vi "Robotics Environment Simulator.vi"() -> ()   [LabVIEW 2011]
doc: "This VI starts and stops the environment simulator and serves as the master VI for your simulation code. Open and run this VI to display the environment simulator, or open the block diagram to view or modify simulation code."
uses:
  <vilib>/robotics/Simulator/NI_Robotics_Simulator.lvlib
panel:
  in  "manifest filename":string="Robotics Environment Simulator.xml"
  in  "stop":bool
  # "* Press the Run button to display the Robotics Environment Simulator.\n* Select Window>>Show Block Diagram or press <Ctrl-E> to view the block diagram, where you can add or modify simulation code. Add controls and indicators to the front panel of this VI to pass data into and out of the simulation code.\n* The manifest file must exist in same directory as the .lvproj file."
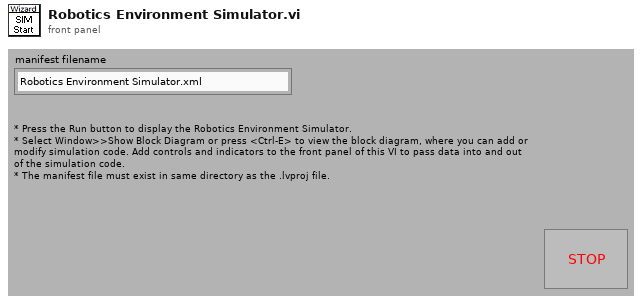
[diagram p1: front panel]
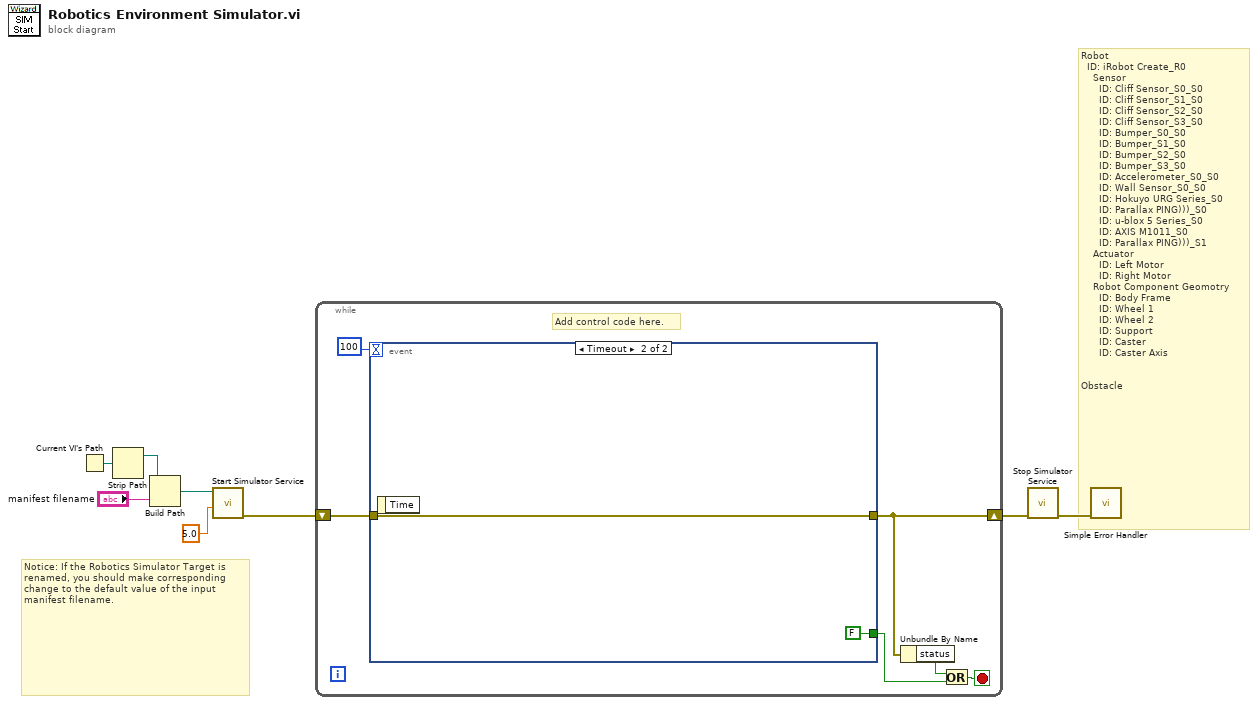
[diagram p0: block diagram]
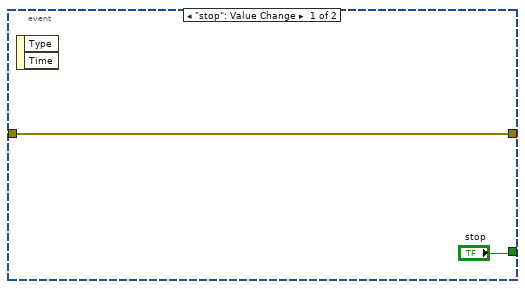
[diagram p2: hidden frame]
diagram:
  # "Robot\n\t\tID: iRobot Create_R0\n\t\t\t\tSensor\n\t\t\t\t\t\tID: Cliff Sensor_S0_S0\n\t\t\t\t\t\tID: Cliff Sensor_S1_S0\n\t\t\t\t\t\tID: Cliff Sensor_S2_S0\n\t\t\t\t\t\tID: Cliff Sensor_S3_S0\n\t\t\t\t\t\tID: Bumper_S0_S0\n\t\t\t\t\t\tID: Bumper_S1_S0\n\t\t\t\t\t\tID: Bumper_S2_S0\n\t\t\t\t\t\tID: Bumper_S3_S0\n\t\t\t\t\t\tID: Accelerometer_S0_S0\n\t\t\t\t\t\tID: Wall Sensor_S0_S0\n\t\t\t\t\t\tID: Hokuyo URG Series_S0\n\t\t\t\t\t\tID: Parallax PING)))_S0\n\t\t\t\t\t\tID: u-blox 5 Series_S0\n\t\t\t\t\t\tID: AXIS M1011_S0\n\t\t\t\t\t\tID: Parallax PING)))_S1\n\t\t\t\tActuator\n\t\t\t\t\t\tID: Left Motor\n\t\t\t\t\t\tID: Right Motor\n\t\t\t\tRobot Component Geomotry\n\t\t\t\t\t\tID: Body Frame\n\t\t\t\t\t\tID: Wheel 1\n\t\t\t\t\t\tID: Wheel 2\n\t\t\t\t\t\tID: Support\n\t\t\t\t\t\tID: Caster\n\t\t\t\t\t\tID: Caster Axis\n\n\nObstacle"
  # "Notice: If the Robotics Simulator Target is renamed, you should make corresponding change to the default value of the input manifest filename."
  n1 = Current VI's Path() -> (path=w6:path)
  n2 = Strip Path(path=w6) -> (stripped path=w5:path)  [unwired: 1 out]
  n3 = Build Path(base path=w5, name or relative path="manifest filename") -> (appended path=w4:path)
  n4 = call <vilib>:"Start Simulator Service.vi"("step size (ms)"=5.0 ("stepsize(ms)"), "manifest file"=w4) -> ("error out"=w1:errorcluster)  [unwired: 9 in]
  n5 = while {
    shift-right: [w10] -> w7
    shift-left: w1 -> [w13]
    stop <- w11 stop-if-true
    # "Add control code here."
    n6 = event shown="[1] Timeout" {
      selector: _ -> [_ _]
      dyn-events: _ -> [_ _]
      timeout: 100 -> [_ _]
      tunnel: ["stop" FALSE ("stop")] -> w12
      tunnel: [w15 w18] -> w10
      tunnel: w13 -> [w15 w18]
      event "stop": Value Change {
        n7 = event-data() -> ()  [unwired: 1 in, 2 out]
      }
      event Timeout {
        n8 = event-data() -> ()  [unwired: 1 in, 1 out]
      }
    }
    n9 = Unbundle By Name(w10) -> ("status"=w9:bool)
    n10 = Or(x=w9, y=w12) -> (x .or. y?=w11:bool)
  }
  n11 = call <vilib>:"Stop Simulator Service.vi"("error in (no error)"=w7) -> ("error out"=w2:errorcluster)  [unwired: 10 in]
  n12 = call <vilib>:"Simple Error Handler.vi"("error in (no error)"=w2) -> ()  [unwired: 4 in, 5 out]
